vi "RDS Serial Handle Frame.vi"(8 "error in (no error)":errorcluster, 10 "RDS Serial Frame":refnum<class "RDS Serial Frame.lvclass">, 11 "GPS Instrument in":refnum<class "GPS Instrument.lvclass">) -> (0 "error out":errorcluster, 3 "GPS Instrument out":refnum<class "GPS Instrument.lvclass">)   [LabVIEW 2015, in "GPS Instrument.lvlib" / "GPS Instrument.lvclass"]
uses:
  GPS Instrument.lvclass
  Libraries/RDS Serial Handler/RDS Serial Frame.lvclass
  Libraries/RDS Serial Handler/RDS Serial Frame.lvclass/RDS Serial Frame.ctl
  Libraries/RDS Child Messages/GPS Data Message/GPS Data Message.lvclass
  Libraries/RDS Framework/RDS Message ID.ctl
  Libraries/RDS Framework/RDS Message Class/RDS Message.lvclass/RDS Message.ctl
  Libraries/RDS Child Messages/GPS Data Message/GPS Data Message.lvclass/GPS Data Message.ctl
  Libraries/3rd Party/NMEA_GPS/NMEA.lvlib
  Libraries/RDS Framework/RDS Message Class/RDS Message.lvclass
  Actors/RDS Parent Actor/RDS Parent Actor/RDS Parent Actor.lvclass
  Libraries/RDS Child Messages/RDS Child Messages.lvlib
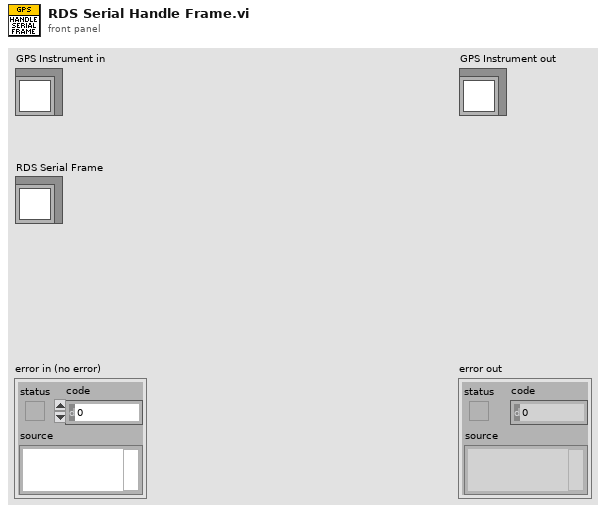
[diagram p1: front panel]
types:
  T1 = typedef "RDS Child Messages.lvlib/RDS Message ID.ctl" = enum16{"RDS Hello World", "String Message", "AIP_Status", "AIP_Command", "GPS_Data", "MCB_Command", "MCB_Status", "Compass_Data", "Depth_Data", "Battery_Data", "Contoller_State", "Set_Mag_Dev", "BTB_Shutdown", "State_Sample_Request", "State_Sample", "PID_Gains_Set", "Helm_Limiter_Set", "Helm_Heading_Command", "Helm_Steering_Command", "Helm_Status", "Controller_Message", "AIP_Set_Min_Depth", "Mission_Controller_State", "Mission_Upload", "Mission_Set_Op_and_Run", "Mission_Settings_Set"}
  T2 = typedef "RDS Libraries.lvlib/NMEA.lvlib/NMEA_GPRMC-data.ctl" = cluster{"TimeStamp":timestamp, "Validity":bool, "Latitude":dbl, "Latitude-Direction":T3, "Longitude":dbl, "Longitude-Direction":T4, "Speed in knots":sgl, "True course":sgl, "Date Stamp":timestamp, "Magnetic Variation (East/West)":sgl, "GPS Latitude":dbl, "GPS Longitude":dbl}
  T3 = typedef "RDS Libraries.lvlib/NMEA.lvlib/NMEA_LatitudeDirection.ctl" = enum16{"", "North", "South"}
  T4 = typedef "RDS Libraries.lvlib/NMEA.lvlib/NMEA_LongitudeDirection.ctl" = enum16{"", "East", "West"}
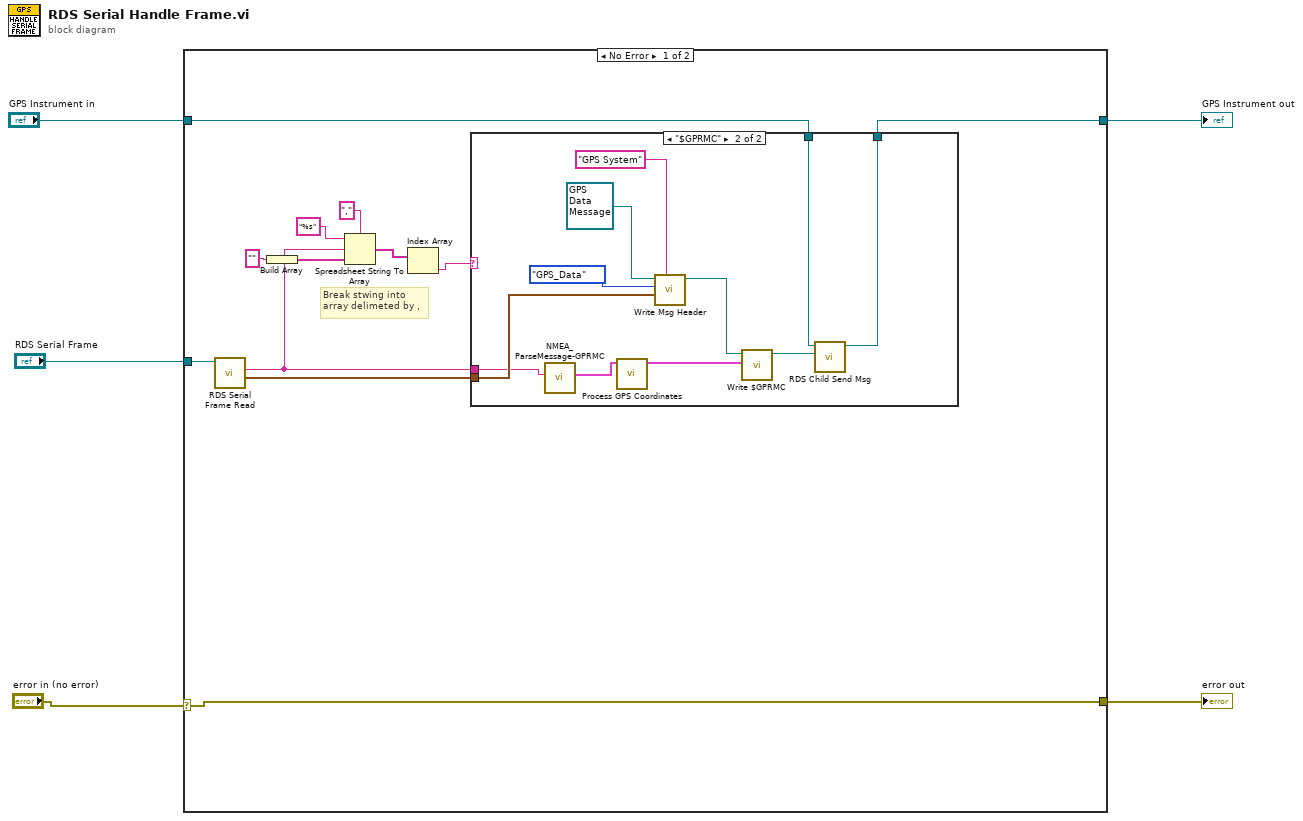
[diagram p0: block diagram]
diagram:
  n1 = case shown="No Error" "error in (no error)" {
    selector: "error in (no error)" -> [w17 w31]
    tunnel: [w17 w31] -> w4
    tunnel: [w13 w30] -> w3
    tunnel: "GPS Instrument in" -> [w14 w30]
    tunnel: "RDS Serial Frame" -> [w16 _]
    frame No Error {
      # "Break stwing into\narray delimeted by ,"
      n2 = call "RDS Serial Frame Read.vi"("RDS Serial Frame in"=w16) -> ("Time Stamp"=w15:timestamp, "Serial String"=w7:string)  [unwired: 7 in, 2 out]
      n3 = Build Array("") -> (w10:string[])
      n4 = Spreadsheet String To Array(delimiter (Tab)=",", format string="%s", spreadsheet string=w7, array type (2D Dbl)=w10) -> (array=w8:string[])
      n5 = Index Array(array=w8) -> (element=w6:string)  [unwired: 1 in]
      n6 = case shown="\"$GPRMC\"" w6 {
        tunnel: w15 -> [_ w29]
        tunnel: w14 -> [w18 w24]
        tunnel: [w18 w23] -> w13
        tunnel: w7 -> [_ w21]
        frame "False", Default {
        }
        frame "$GPRMC" {
          n7 = call "NMEA_ParseMessage-GPRMC.vi"("$GPRMC-message_IN"=w21) -> ("$GPRMC-message_OUT"=w20:T2)  [unwired: 9 in, 1 out]
          n8 = call "Process GPS Coordinates.vi"("GPRMC-data"=w20) -> ("GPRMC Data"=w19:T2)  [unwired: 10 in]
          n9 = call "Write Msg Header.vi"("Sender Name"="GPS System", "Time Stamp"=w29, "Msg ID"=RDS_Message_ID."GPS_Data", "RDS Message in"=refnum<class "GPS Data Message.lvclass"> refnum ("RDS Child Messages.lvlib:GPS Data Message.lvclass")) -> ("RDS Message out"=w27:refnum<class "GPS Data Message.lvclass">)  [unwired: 6 in, 1 out]
          n10 = call "Write $GPRMC.vi"("GPRMC-data"=w19, "GPS Data Message in"=w27) -> ("GPS Data Message out"=w25:refnum<class "GPS Data Message.lvclass">)  [unwired: 8 in, 1 out]
          n11 = call "RDS Child Send Msg.vi"("RDS Message"=w25, "RDS Parent Actor in"=w24) -> ("RDS Parent Actor out"=w23:refnum<class "GPS Instrument.lvclass">)  [unwired: 8 in, 1 out]
        }
      }
    }
    frame Error {
    }
  }
  "error out" <- w4
  "GPS Instrument out" <- w3
